vi "RT_TestDalayWithReentrant.vi"() -> ()   [LabVIEW 2010]
panel:
  in  "Time Target":dbl=50.0
  out "Numeric":dbl
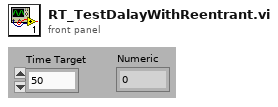
[diagram p1: front panel]
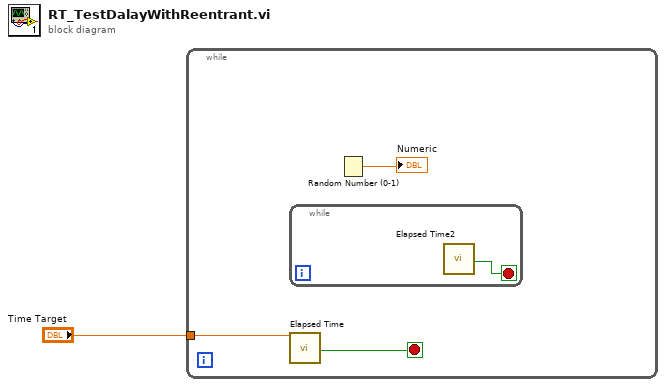
[diagram p0: block diagram]
diagram:
  n1 = while {
    tunnel: "Time Target" -> [w2]
    stop <- w4 stop-if-true
    n2 = while {
      stop <- w5 stop-if-true
      n3 = call "Elapsed Time2"() -> ("Time has Elapsed"=w5:bool)  [unwired: 12 in, 7 out]
    }
    n4 = call "Elapsed Time"("Time Target (s)"=w2) -> ("Time has Elapsed"=w4:bool)  [unwired: 11 in, 7 out]
    n5 = Random Number (0-1)() -> (number: 0 to 1=→"Numeric":dbl)
  }
